vi "Get Tx Queue Status Section and Channels.vi"(8 "error in":errorcluster, 11 "Custom Device Ref in":T1 format="%.0x") -> (0 "error out":errorcluster, 1 "Tx Queue Status channel Refs":T1[](array[typedef]) format="%.0x", 2 "Tx Queue Status Section Ref out":T1 format="%.0x", 3 "Custom Device Ref out":T1 format="%.0x", 4 "Found?":bool)   [LabVIEW 2020, in "afdx_custom_device Scripting.lvlib"]
uses:
  afdx_custom_device Scripting.lvlib
  <vilib>/NI VeriStand/Custom Device API/Custom Device Item Ref.ctl
  Constants.vi
  <vilib>/NI VeriStand/Custom Device Tools/Custom Device Utility Library/NI VeriStand - Search for Item by GUID.vi
  <vilib>/NI VeriStand/Custom Device Tools/Custom Device Utility Library/NI VeriStand - Search for Item by Name.vi
  <vilib>/NI VeriStand/Custom Device Tools/Custom Device Utility Library/Custom Device Utility Library.lvlib
  <vilib>/NI VeriStand/Custom Device API/Custom Device API.lvlib
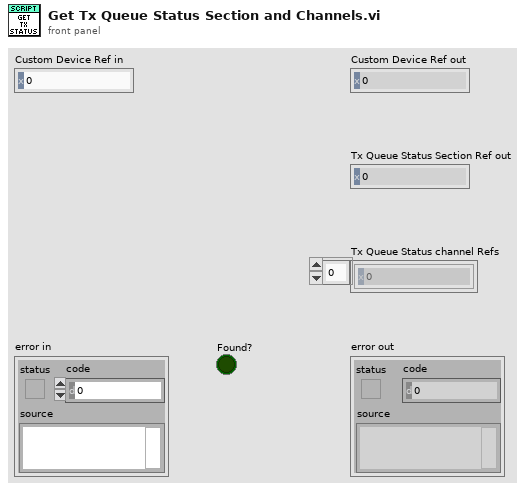
[diagram p1: front panel]
types:
  T1 = typedef "Custom Device API.lvlib/Custom Device Item Ref.ctl" = u64
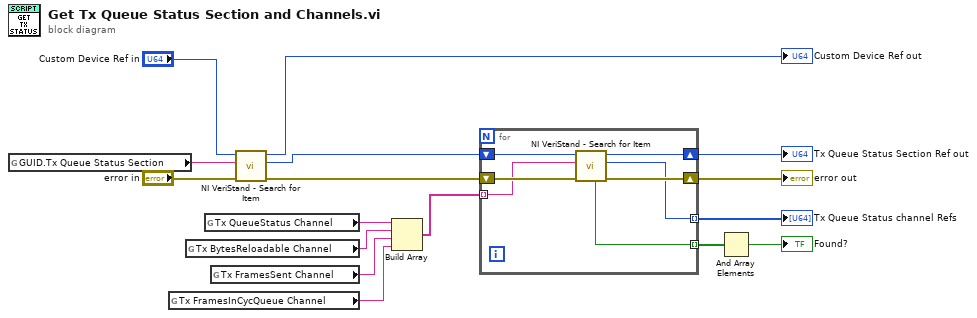
[diagram p0: block diagram]
diagram:
  n1 = global read "Constants.vi" "GUID.Tx Queue Status Section"() -> (w13:string)
  n2 = global read "Constants.vi" "Tx FramesInCycQueue Channel"() -> (w4:string)
  n3 = global read "Constants.vi" "Tx BytesReloadable Channel"() -> (w6:string)
  n4 = global read "Constants.vi" "Tx QueueStatus Channel"() -> (w7:string)
  n5 = global read "Constants.vi" "Tx FramesSent Channel"() -> (w5:string)
  n6 = call-poly <vilib>:"NI VeriStand - Search for Item.vi"("error in"="error in", "Item GUID"=w13, "Section Ref in"="Custom Device Ref in") -> ("error out"=w14:errorcluster, "Item Ref"=w11:T1, "Section Ref out"=→"Custom Device Ref out":T1)  [unwired: 5 in, 1 out]
  n7 = Build Array(w7, w6, w5, w4) -> (w3:string[])
  n8 = for {
    tunnel: [w19] -> w8 mode=indexing
    shift-right: [w20] -> w9
    shift-left: w14 -> [w23]
    tunnel: w3 -> [w18] mode=indexing
    shift-right: [w22] -> w12
    shift-left: w11 -> [w21]
    tunnel: [w17] -> w2 mode=indexing
    n9 = call-poly <vilib>:"NI VeriStand - Search for Item.vi"("error in"=w23, "Item Name"=w18, "Section Ref in"=w21) -> ("error out"=w20:errorcluster, "Item Ref"=w19:T1, "Section Ref out"=w22:T1, "Found"=w17:bool)  [unwired: 5 in]
  }
  "Tx Queue Status Section Ref out" <- w12
  "error out" <- w9
  "Tx Queue Status channel Refs" <- w8
  n10 = And Array Elements(Boolean array=w2) -> (logical AND=→"Found?":bool)
